vi "Main.vi"(8 "error in":errorcluster caption="entrée d'erreur") -> (0 "error out":errorcluster caption="sortie d'erreur")   [LabVIEW 2026]
uses:
  <vilib>/DAQmx/read.llb/DAQmx Read (Analog 1D DBL 1Chan NSamp).vi
  <vilib>/DAQmx/read.llb/DAQmx Read (Counter 1D DBL 1Chan NSamp).vi
  <vilib>/DAQmx/miscellaneous.llb/DAQmx Fill In Error Info.vi
panel:
  in  "Dwell time (µs)":dbl=2.0 format="%#_13g"
  out "PMT_Scan":dbl[][](graph)
  out "PMT_i(t)":dbl[](graph)
  out "APD_i(t)":dbl[](graph)
  out "APD_Scan":dbl[][](graph)
  in  "Stop":bool
  in  "Continuous?":bool
  in  "Scan XY (T) / i(t) (F)":bool
  in  "Position XY (for i(t))":dbl[](array[numeric])=[5.0, 5.0]
  out "Graphe":dbl[][](graph)
  in  "Scanning cluster":T1={"Nx"=4, "Ny"=4, "# Repetition"=1, "FOV_X (µm)"=100.0, "FOV_Y (µm)"=100.0, "Calib_X"=0.1, "Calib_Y"=0.1, "Center X (µm)"=50.0, "Center_Y (µm)"=50.0, "Bi-directionnal?"=FALSE} {"# Repetition" min=1 step=1; "Ny" min=1 step=1; "Nx" min=1 step=1}
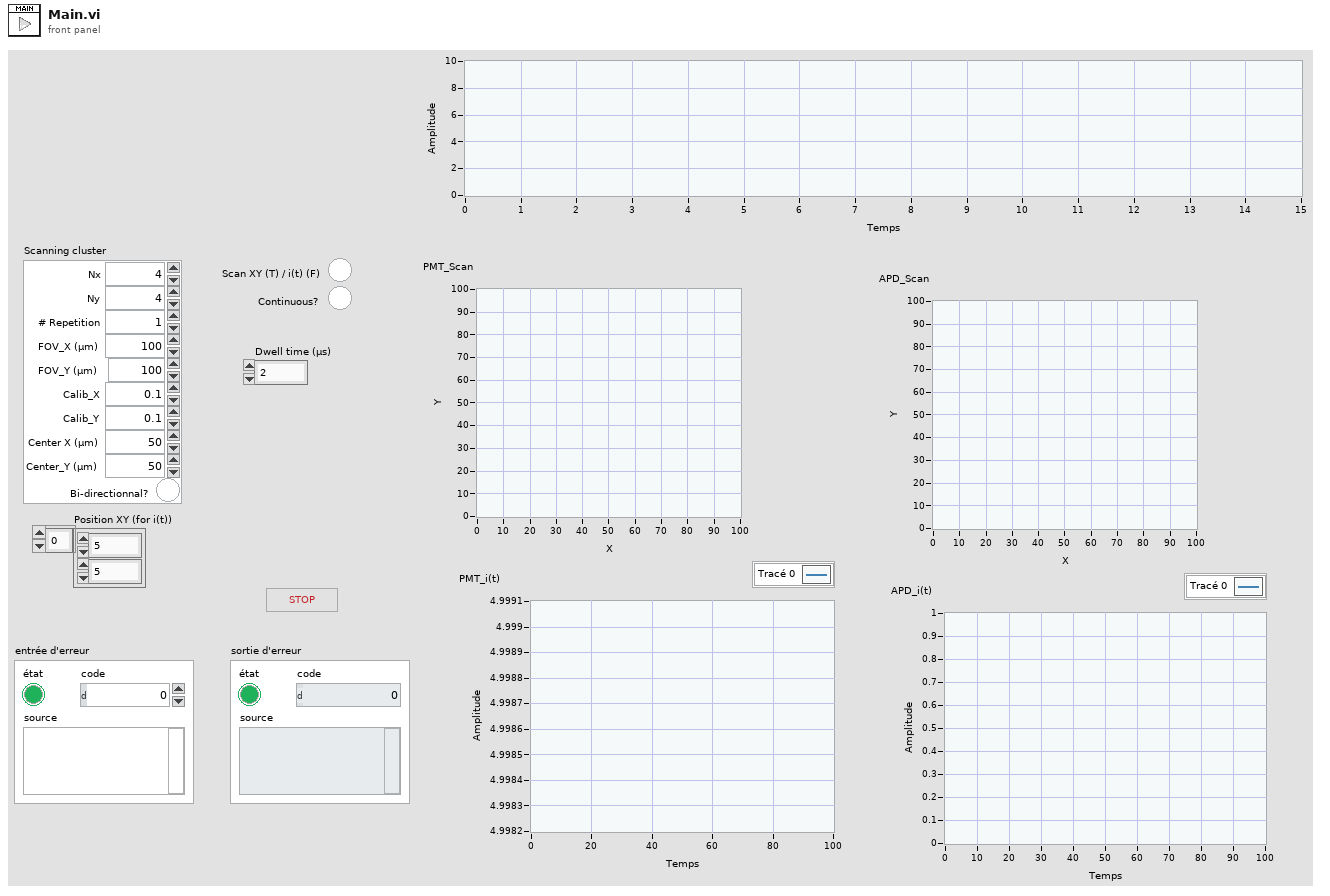
[diagram p1: front panel]
types:
  T1 = cluster{"Nx":u16, "Ny":u16, "# Repetition":u16, "FOV_X (µm)":dbl, "FOV_Y (µm)":dbl, "Calib_X":dbl, "Calib_Y":dbl, "Center X (µm)":dbl, "Center_Y (µm)":dbl, "Bi-directionnal?":bool}
  T2 = cluster{"CO task":refnum<k21>, "AO task":refnum<k21>, "AI task":refnum<k21>, "CI task":refnum<k21>}
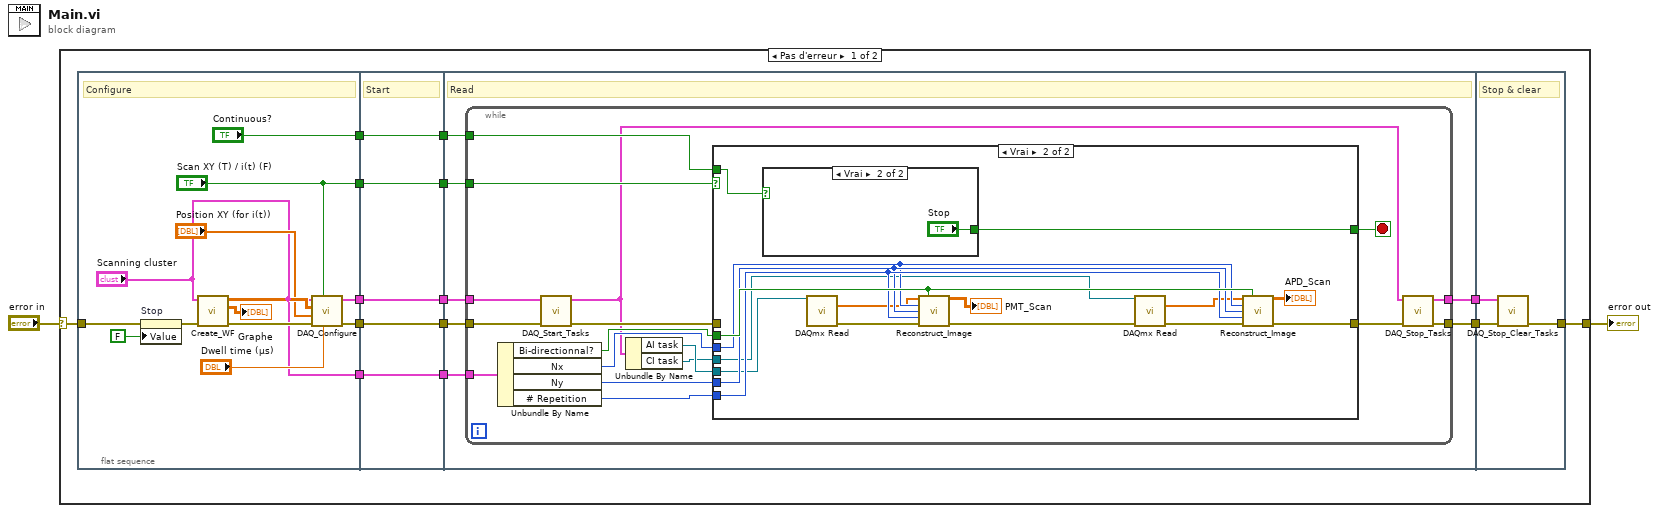
[diagram p0: block diagram]
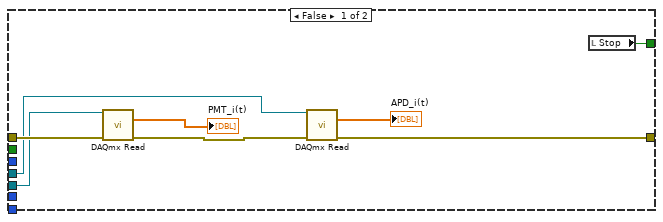
[diagram p2: hidden frame]
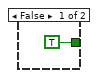
[diagram p3: hidden frame]
diagram:
  n1 = case shown="Pas d'erreur" "error in" {
    selector: "error in" -> [w16 w88]
    tunnel: [w4 w88] -> w1
    frame No Error {
      n2 = flat-sequence {
        tunnel: w16 -> [w19]
        tunnel: [w28] -> w15
        tunnel: [w23] -> w13
        tunnel: ["Scan XY (T) / i(t) (F)"] -> w12
        tunnel: ["Scanning cluster"] -> w8
        tunnel: ["Continuous?"] -> w6
        tunnel: w15 -> [w31]
        tunnel: [w31] -> w14
        tunnel: w13 -> [w30]
        tunnel: w12 -> [w34]
        tunnel: [w34] -> w11
        tunnel: [w30] -> w10
        tunnel: [w33] -> w9
        tunnel: w8 -> [w33]
        tunnel: [w32] -> w7
        tunnel: w6 -> [w32]
        tunnel: w14 -> [w41]
        tunnel: w11 -> [w40]
        tunnel: w10 -> [w39]
        tunnel: w9 -> [w38]
        tunnel: w7 -> [w37]
        tunnel: [w36] -> w5
        tunnel: [w35] -> w3
        tunnel: w5 -> [w86]
        tunnel: [w87] -> w4
        tunnel: w3 -> [w85]
        frame #0 {
          # "Configure"
          n3 = property on="Stop" class="Bool (strict)"(error in=w19, "Value"=FALSE ("Stop")) -> (error out=w18:errorcluster)  [unwired: 1 in, 1 out]
          n4 = call "Create_WF.vi"("error in"=w18, "Scanning cluster"="Scanning cluster") -> ("error out"=w29:errorcluster, "Graphe"=→"Graphe":dbl[][], "Scanning positions"=w27:dbl[][])  [unwired: 7 in]
          n5 = call "DAQ_Configure.vi"("Dwell time (µs)"="Dwell time (µs)", "Scan XY (T) / i(t) (F)"="Scan XY (T) / i(t) (F)", "error in"=w29, "Position XY (for i(t))"="Position XY (for i(t))", "Scanning positions"=w27, "Scanning cluster"="Scanning cluster") -> ("error out"=w28:errorcluster, "Task cluster"=w23:T2)  [unwired: 4 in]
        }
        frame #1 {
          # "Start"
        }
        frame #2 {
          # "Read"
          n6 = while {
            tunnel: w41 -> [w50]
            tunnel: w40 -> [w58]
            tunnel: w39 -> [w49]
            tunnel: w38 -> [w57]
            tunnel: w37 -> [w52]
            tunnel: [w44] -> w36
            tunnel: [w43] -> w35
            stop <- w51 stop-if-true
            n7 = Unbundle By Name(w57) -> ("Bi-directionnal?"=w56:bool, "Nx"=w55:u16, "Ny"=w54:u16, "# Repetition"=w53:u16)
            n8 = call "DAQ_Start_Tasks.vi"("entrée d'erreur (pas d'erreur)"=w50, "Task cluster"=w49) -> ("sortie d'erreur"=w48:errorcluster, "Task cluster OUT"=w42:T2)  [unwired: 8 in]
            n9 = Unbundle By Name(w42) -> ("AI task"=w47:refnum<k21>, "CI task"=w46:refnum<k21>)
            n10 = case shown="Vrai" w58 {
              tunnel: w56 -> [_ w79]
              tunnel: w55 -> [_ w76]
              tunnel: w54 -> [_ w77]
              tunnel: w53 -> [_ w78]
              tunnel: w52 -> [_ w82]
              tunnel: [w63 w81] -> w51
              tunnel: [w64 w71] -> w45
              tunnel: w48 -> [w61 _]
              tunnel: w47 -> [w60 w68]
              tunnel: w46 -> [w59 w67]
              frame False {
                n11 = call-poly <vilib>:"DAQmx Read.vi"("task/channels in"=w60, "error in"=w61) -> ("data"=→"PMT_i(t)":dbl[], "error out"=w66:errorcluster)  [unwired: 11 in, 1 out]
                n12 = call-poly <vilib>:"DAQmx Read.vi"("task/channels in"=w59, "error in"=w66) -> ("data"=→"APD_i(t)":dbl[], "error out"=w64:errorcluster)  [unwired: 11 in, 1 out]
                n13 = local read "Stop"() -> (w63:bool)
              }
              frame True {
                n14 = case shown="Vrai" w82 {
                  tunnel: [TRUE ("Stop") "Stop"] -> w81
                  frame False {
                  }
                  frame True {
                  }
                }
                n15 = call-poly <vilib>:"DAQmx Read.vi"("task/channels in"=w68) -> ("data"=w74:dbl[], "error out"=w75:errorcluster)  [unwired: 12 in, 1 out]
                n16 = call "Reconstruct_Image.vi"("Data_AI"=w74, "Bidirectionnel?"=w79, "Nx"=w76, "Ny"=w77, "# Repetition"=w78, "error in"=w75) -> ("Channel 1"=→"PMT_Scan":dbl[][], "error out"=w80:errorcluster)  [unwired: 7 in, 1 out]
                n17 = call-poly <vilib>:"DAQmx Read.vi"("task/channels in"=w67, "error in"=w80) -> ("data"=w73:dbl[], "error out"=w72:errorcluster)  [unwired: 11 in, 1 out]
                n18 = call "Reconstruct_Image.vi"("Data_AI"=w73, "Bidirectionnel?"=w79, "Nx"=w76, "Ny"=w77, "# Repetition"=w78, "error in"=w72) -> ("Channel 1"=→"APD_Scan":dbl[][], "error out"=w71:errorcluster)  [unwired: 7 in, 1 out]
              }
            }
            n19 = call "DAQ_Stop_Tasks.vi"("error in"=w45, "Cluster tasks"=w42) -> ("error out"=w44:errorcluster, "Cluster tasks OUT"=w43:T2)  [unwired: 8 in]
          }
        }
        frame #3 {
          # "Stop & clear"
          n20 = call "DAQ_Stop_Clear_Tasks.vi"("error in"=w86, "Cluster tasks"=w85) -> ("sortie d'erreur"=w87:errorcluster)  [unwired: 9 in]
        }
      }
    }
    frame Error {
    }
  }
  "error out" <- w1
